vi "SRV_Get Enum Info.vi"(6 "Enum type string":i16[](array[numeric])) -> (0 "Enum Strings":string[](array[string]), 2 "Enum Size":i32, 3 "Enum Name":string)   [LabVIEW 2014]
doc: "<B>Use \"SRV_Get Enum Info (Variant Input).vi\" instead of this VI in conjunction with \"Variant to Flattened String\" function.</B>\n\n<B>Function Description:</B> Returns information about an enumerated type.\nUse LabVIEW's \"Variant to Flattened String\" function on the enum and wire the \"type string\" output into this VI.\n\n<B>Inputs:</B>\nEnum type string (1-D array of word integer):\ncontains the binary type descriptor for the enumerated type\n \n<B>Outputs:</B>\nEnum Name (string):\n\nEnum Size (long integer):\n\nEnum Strings (1-D array of string):\n\n<B>User Guide:</B> Use LabVIEW's \"Variant to Flattened String\" function on the enum and wire the \"type string\" output into this VI.\n\"Flatten To String\" can be found on the Functions palette >> Advanced >> Data Manipulation.\n\n<B>Note:</B> Type string code values might change in future LabVIEW versions. This version of the VI works for:\nLabVIEW 5.1.1, LabVIEW 6.0.2, LabVIEW 7.x, LabVIEW 8.x, LabVIEW 9.x (moving from 'Flatten to String' to 'Variant to Flattened String')\n\n<B>Keywords:</B> enum, enumerated type\n\n<B>Initial Developer:</B> Mike Schultz"
panel:
  # "Use \"SRV_Get Enum Info (Variant Input).vi\" instead of this VI in conjunction with \"Variant to Flattened String\" function."
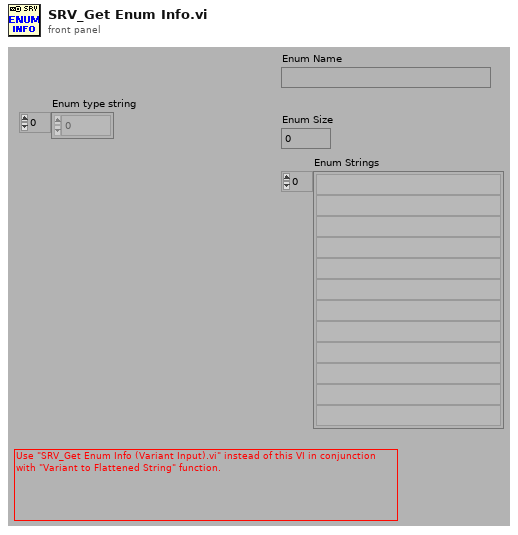
[diagram p1: front panel]
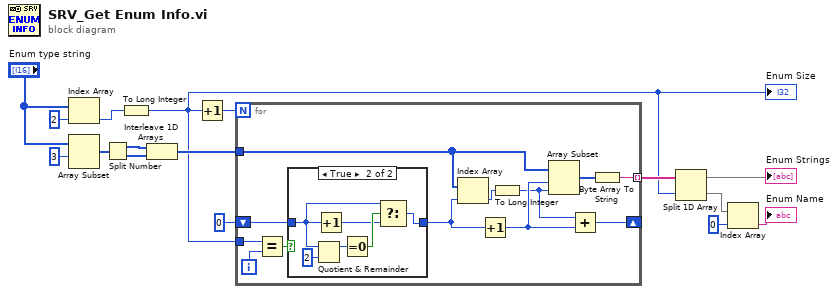
[diagram p0: block diagram]
diagram:
  n1 = Index Array(array="Enum type string", index=2 ("Index")) -> (element=w9:i16)
  n2 = Array Subset(array="Enum type string", index=3 ("Array Index")) -> (w2:i16[])  [unwired: 1 in]
  n3 = Split Number(x=w2) -> (hi(x)=w14:u8[], lo(x)=w13:u8[])
  n4 = To Long Integer(number=w9) -> (32bit integer=w1:i32)
  "Enum Size" <- w1
  n5 = Interleave 1D Arrays(w14, w13) -> (w11:u8[])
  n6 = Increment(x=w1) -> (x+1=w10:i32)
  n7 = for {
    N: w10 -> [_]
    tunnel: w11 -> [w27]
    tunnel: [w26] -> w8 mode=indexing
    shift-right: [w23] -> _
    shift-left: 0 ("Index") -> [w18]
    tunnel: w1 -> [w20]
    i -> [w21]
    n8 = Equal?(x=w20, y=w21) -> (x = y?=w19:bool)
    n9 = case shown="True" w19 {
      tunnel: w18 -> [w29 w31]
      tunnel: [w29 w30] -> w17
      frame False {
      }
      frame True {
        n10 = Quotient & Remainder(x=w31, y=2) -> (x-y*floor(x/y)=w34:i32)  [unwired: 1 out]
        n11 = Increment(x=w31) -> (x+1=w32:i32)
        n12 = Equal To 0?(x=w34) -> (x = 0?=w33:bool)
        n13 = Select(t=w31, s=w33, f=w32) -> (s? t:f=w30:i32)
      }
    }
    n14 = Index Array(array=w27, index=w17) -> (element=w25:u8)
    n15 = Increment(x=w17) -> (x+1=w24:i32)
    n16 = To Long Integer(number=w25) -> (32bit integer=w22:i32)
    n17 = Array Subset(array=w27, index=w24, length=w22) -> (w28:u8[])
    n18 = Add(x=w22, y=w24) -> (x+y=w23:i32)
    n19 = Byte Array To String(unsigned byte array=w28) -> (string=w26:string)
  }
  n20 = Split 1D Array(array=w8, index=w1) -> (first subarray=→"Enum Strings":string[], second subarray=w6:string[])
  n21 = Index Array(array=w6, index=0 ("Index")) -> (element=→"Enum Name":string)
